vi "Obtain Queue.vi"(8 "error in (no error)":errorcluster, 9 "Depth":i32, 11 "Connection in":refnum<class "Connection.lvclass">) -> (0 "error out":errorcluster, 2 "Queue":refnum<queue>, 3 "Connection out":refnum<class "Connection.lvclass">)   [LabVIEW 2020, in "Connection.lvclass"]
uses:
  Connection.lvclass
  Connection.lvclass/Connection.ctl
  Element.ctl
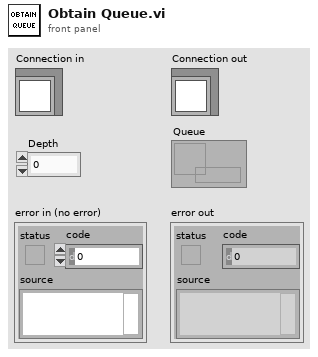
[diagram p1: front panel]
types:
  T1 = typedef "Connection.lvclass/Element.ctl" = dbl
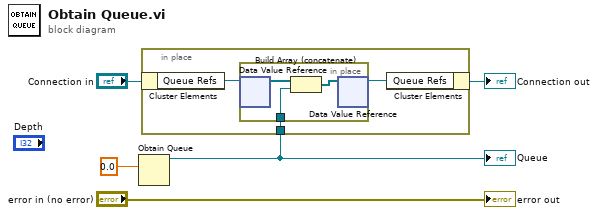
[diagram p0: block diagram]
diagram:
  n1 = Obtain Queue(element data type=T1 0.0 ("Element")) -> (queue out=w2:refnum<queue>)  [unwired: 4 in, 2 out]
  "Queue" <- w2
  n2 = in-place {
    in-place-border: w2 -> [w6]
    n3 = in-place-cluster #1("Connection in") -> ("Queue Refs"=w8:refnum<data-value>)
    n4 = in-place {
      in-place-border: w6 -> [w10]
      n5 = in-place-dvr #2(w8) -> (w11:refnum<queue>[])  [unwired: 1 out]
      n6 = Build Array (concatenate)(w11, w10) -> (w9:refnum<queue>[])
      n7 = in-place-dvr #2(w9) -> (w7:refnum<data-value>)  [unwired: 1 out]
    }
    n8 = in-place-cluster #1("Queue Refs"=w7) -> (→"Connection out":refnum<class "Connection.lvclass">)
  }
  "error out" <- "error in (no error)"
